vi "SFPBlock Processing Loop State Manager.vi"(8 "error in":errorcluster, 9 "variant":variant, 10 "message in":string, 11 "Message Queue":refnum<queue>) -> (0 "error out":errorcluster, 1 "duplicate variant":variant, 2 "message out":string, 3 "duplicate Message Queue":refnum<queue>)   [LabVIEW 2024, in "DSA_CFG_ACQ.lvlib"]
uses:
  DSA_CFG_ACQ.lvlib
  controls/SFPBlock Processing States.ctl
  Dynamic Signal Acquisition (Interactive).lvlib
  8ab9d2bb-6bd8-408b-a319-3e4023a23bad.vi
  Message Queue/Message Cluster.ctl
  Message Queue/SFPMessage Queue.lvlib
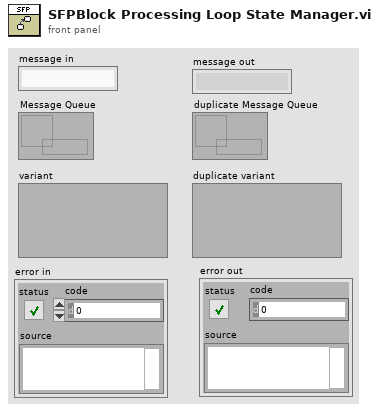
[diagram p1: front panel]
types:
  T1 = typedef "Dynamic Signal Acquisition (Interactive).lvlib/SFPBlock Processing States.ctl" = enum16{"No Error", "Error"}
  T2 = typedef "SFPBlock Processing States.ctl" = enum16{"No Error", "Error"}
  T3 = typedef "DSA_CFG_ACQ.lvlib/SFPMessage Queue.lvlib/Message Cluster.ctl" = cluster{"Message":string, "Message Data":variant}
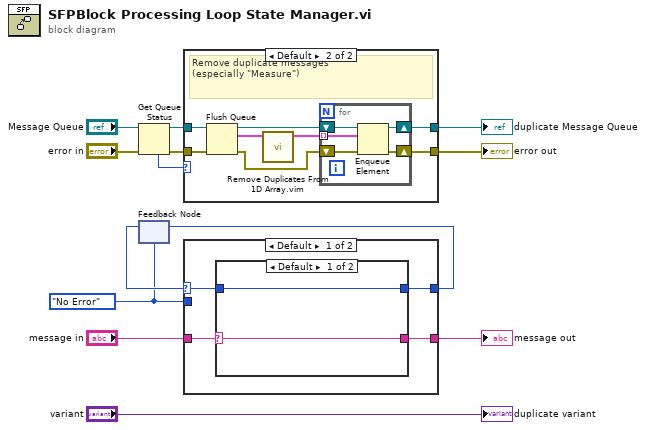
[diagram p0: block diagram]
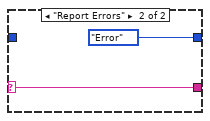
[diagram p3: hidden frame]
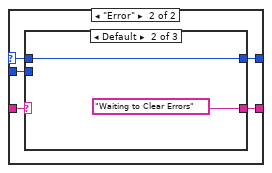
[diagram p4: hidden frame]
diagram:
  w8 = SFPBlock_Processing_States."No Error" ("State")
  n1 = Get Queue Status(queue="Message Queue", error in (no error)="error in") -> (queue out=w3:refnum<queue>, error out=w1:errorcluster, # elements in queue=w5:i32)  [unwired: 1 in, 5 out]
  n2 = feedback #1(w8) -> (w10:T2)
  n3 = case shown="Default" w5 {
    tunnel: [w15 w18] -> w4
    tunnel: w3 -> [w15 w23]
    tunnel: [w14 w16] -> w2
    tunnel: w1 -> [w14 w21]
    frame 0..7 {
      # "number of elements < 8"
    }
    frame Default {
      # "Remove duplicate messages \n(especially \"Measure\")"
      n4 = Flush Queue(queue=w23, error in (no error)=w21) -> (queue out=w22:refnum<queue>, remaining elements=w20:T3[], error out=w17:errorcluster)
      n5 = call "Remove Duplicates From 1D Array.vim"("array"=w20) -> ("array with duplicates removed"=w19:T3[])  [unwired: 10 in]
      n6 = for {
        tunnel: w19 -> [w27] mode=indexing
        shift-right: [w26] -> w18
        shift-left: w22 -> [w28]
        shift-right: [w24] -> w16
        shift-left: w17 -> [w25]
        n7 = Enqueue Element(queue=w28, element=w27, error in (no error)=w25) -> (queue out=w26:refnum<queue>, error out=w24:errorcluster)  [unwired: 1 in, 1 out]
      }
    }
  }
  "duplicate Message Queue" <- w4
  "error out" <- w2
  n8 = case shown="Default" w10 {
    selector: w10 -> [w29 w37]
    tunnel: "message in" -> [w32 w40]
    tunnel: [w31 w41] -> w11
    tunnel: [w30 w38] -> w9
    tunnel: w8 -> [_ w39]
    frame Default {
      n9 = case shown="Default" w32 {
        selector: w32 -> [w34 w36]
        tunnel: [w34 w36] -> w31
        tunnel: [w33 SFPBlock_Processing_States."Error" ("State")] -> w30
        tunnel: w29 -> [w33 _]
        frame Default {
        }
        frame "Report Errors" {
        }
      }
    }
    frame "Error" {
      n10 = case shown="Default" w40 {
        selector: w40 -> [w43 _ w46]
        tunnel: [w43 "Waiting to Clear Errors" w46] -> w41
        tunnel: w39 -> [w42 _ _]
        tunnel: [w42 w44 w47] -> w38
        tunnel: w37 -> [_ w44 w47]
        frame "Error Cleared" {
        }
        frame Default {
        }
        frame "Exit" {
        }
      }
    }
  }
  "message out" <- w11
  n11 = feedback-in #1(w9) -> ()
  "duplicate variant" <- "variant"
